vi "Meas (SubVI).vi"(9 "Param":T1 {"FChB" format="%_4p"; "FChA" format="%_4p"}, 11 "Array in":waveform(dbl)[](array[waveform])) -> (1 "RMS, V":dbl[](array[numeric]), 2 "RMS,mV":dbl[](array[numeric]), 3 "Freq":dbl[](array[numeric]))   [LabVIEW 2017]
uses:
  <vilib>/measure/matone.llb/Extract Single Tone Information 1 Chan.vi
  <vilib>/measure/NI_MAPro.lvlib
panel:
  out "error out":errorcluster
  in  "error in":errorcluster
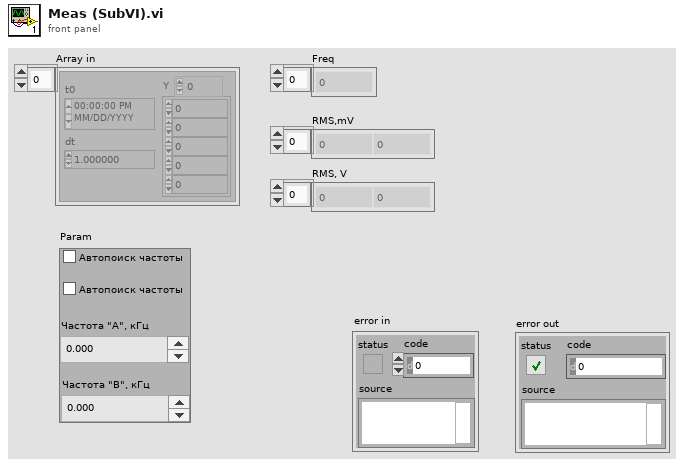
[diagram p1: front panel]
types:
  T1 = cluster{"AutoFindFreqChA":bool, "AutoFindFreqChB":bool, "FChA":dbl, "FChB":dbl}
  T2 = cluster{"approx freq. (optional)":dbl, "search (+/- % of Fsampl.)":dbl}
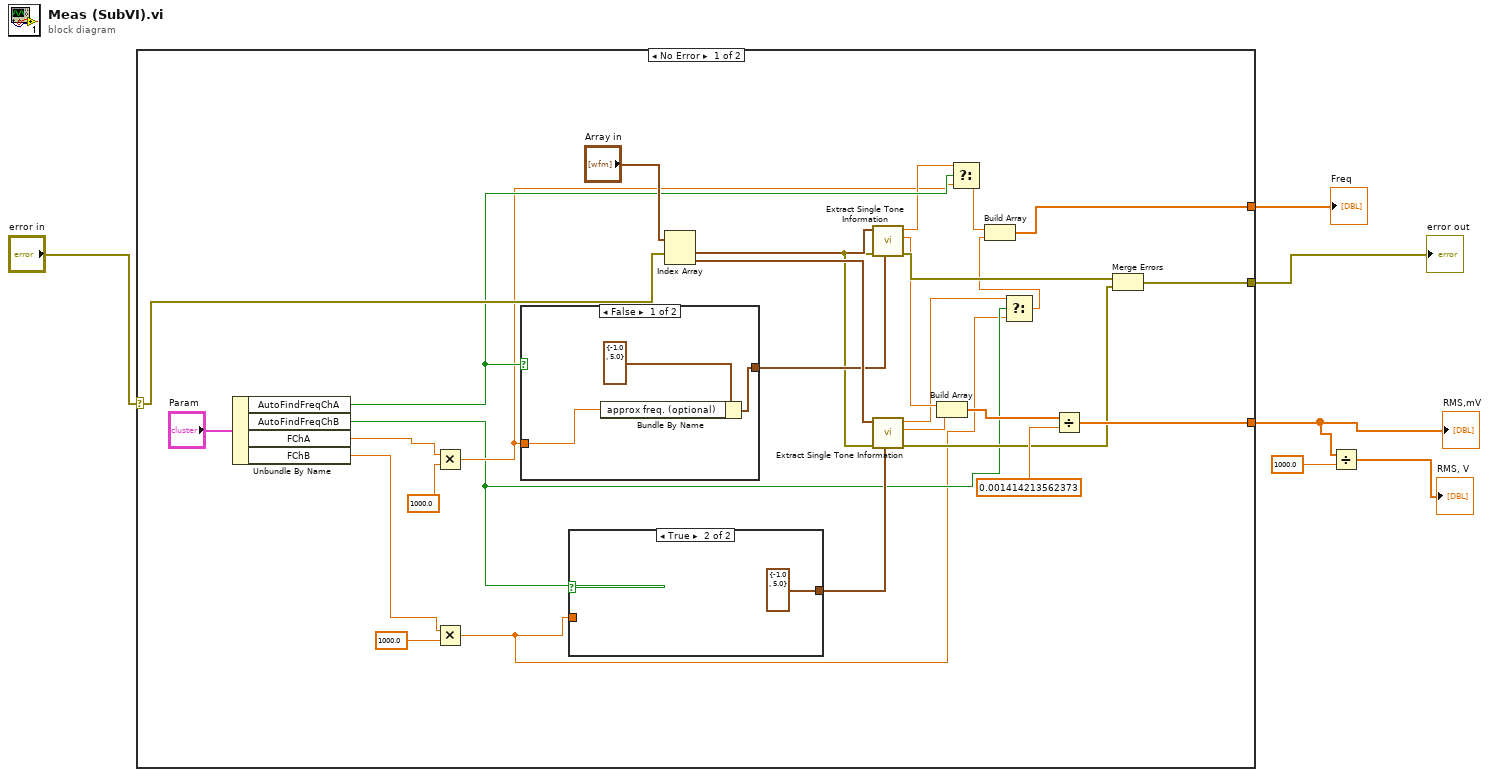
[diagram p0: block diagram]
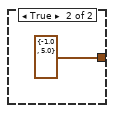
[diagram p2: hidden frame]
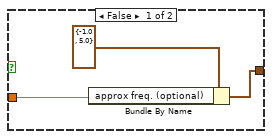
[diagram p3: hidden frame]
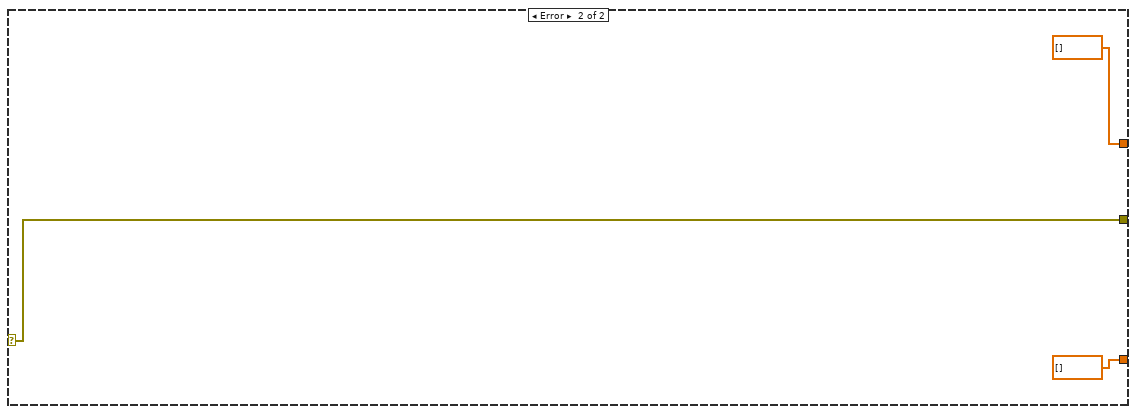
[diagram p4: hidden frame]
diagram:
  n1 = case shown="No Error" "error in" {
    selector: "error in" -> [w21 w45]
    tunnel: [w34 dbl[] []] -> w6
    tunnel: [w28 dbl[] []] -> w2
    tunnel: [w20 w45] -> w4
    frame No Error {
      n2 = Unbundle By Name("Param") -> ("AutoFindFreqChA"=w16:bool, "AutoFindFreqChB"=w11:bool, "FChA"=w19:dbl, "FChB"=w10:dbl)
      n3 = Multiply(x=w19, y=1000.0) -> (x*y=w12:dbl)
      n4 = Multiply(x=w10, y=1000.0) -> (x*y=w7:dbl)
      n5 = case shown="False" w16 {
        tunnel: [w36 T2 {"approx freq. (optional)"=-1.0, "search (+/- % of Fsampl.)"=5.0} ("advanced search")] -> w25
        tunnel: w12 -> [w35 _]
        frame False {
          n6 = Bundle By Name(cluster=T2 {"approx freq. (optional)"=-1.0, "search (+/- % of Fsampl.)"=5.0} ("advanced search"), "approx freq. (optional)"=w35) -> (w36:T2)
        }
        frame True {
        }
      }
      n7 = case shown="True" w11 {
        tunnel: [w40 T2 {"approx freq. (optional)"=-1.0, "search (+/- % of Fsampl.)"=5.0} ("advanced search")] -> w26
        tunnel: w7 -> [w39 _]
        frame False {
          n8 = Bundle By Name(cluster=T2 {"approx freq. (optional)"=-1.0, "search (+/- % of Fsampl.)"=5.0} ("advanced search"), "approx freq. (optional)"=w39) -> (w40:T2)
        }
        frame True {
        }
      }
      n9 = Index Array(array="Array in") -> (element #1=w30:waveform(dbl), element #2=w31:waveform(dbl))  [unwired: 2 in]
      n10 = call-poly <vilib>:"Extract Single Tone Information.vi"("advanced search"=w25, "error in (no error)"=w21, "time signal in"=w30) -> ("error out"=w22:errorcluster, "detected amplitude"=w15:dbl, "detected frequency"=w14:dbl)  [unwired: 3 in, 3 out]
      n11 = call-poly <vilib>:"Extract Single Tone Information.vi"("advanced search"=w26, "error in (no error)"=w21, "time signal in"=w31) -> ("error out"=w23:errorcluster, "detected amplitude"=w32:dbl, "detected frequency"=w9:dbl)  [unwired: 3 in, 3 out]
      n12 = Build Array(w15, w32) -> (w33:dbl[])
      n13 = Select(t=w14, s=w16, f=w12) -> (s? t:f=w13:dbl)
      n14 = Select(t=w9, s=w11, f=w7) -> (s? t:f=w8:dbl)
      n15 = Build Array(w13, w8) -> (w34:dbl[])
      n16 = Divide(x=w33, y=0.001414213562373) -> (x/y=w28:dbl[])
      n17 = Merge Errors(w22, w23) -> (w20:errorcluster)
    }
    frame Error {
    }
  }
  "Freq" <- w6
  "RMS,mV" <- w2
  "error out" <- w4
  n18 = Divide(x=w2, y=1000.0) -> (x/y=→"RMS, V":dbl[])
